vi "Pilot Analyze.vi"(5 "JoystickDevRef":T1) -> (2 "Suction":bool, 3 "x":dbl, 4 "y":dbl, 8 "Canenet L":dbl, 10 "Canenet R":dbl, 13 "Give copilot control rotation":bool, 15 "Slow Drive":bool)   [LabVIEW 2012]
uses:
  <vilib>/Rock Robotics/WPI/Joystick/WPI_JoystickDevRef.ctl
  <vilib>/Rock Robotics/WPI/Joystick/WPI_JoystickDeviceEnum.ctl
panel:
  out "Feeder":bool
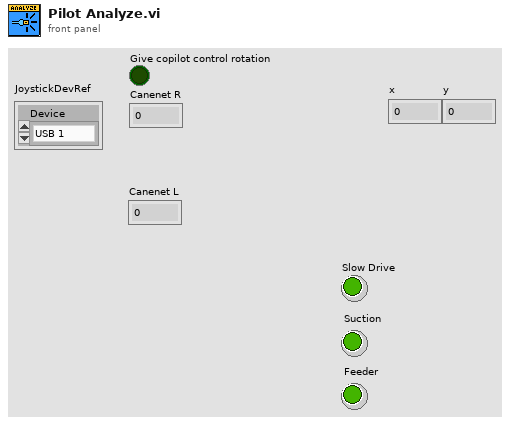
[diagram p1: front panel]
types:
  T1 = typedef "WPI_JoystickDevRef.ctl" = cluster{"Device":T2}
  T2 = typedef "WPI_JoystickDeviceEnum.ctl" = enum16{"USB 1", "USB 2", "USB 3", "USB 4", "Kinect 1", "Kinect 2"}
  T3 = typedef "WPI_JoystickButtonState.ctl" = cluster{"Button 1":bool, "Button 2":bool, "Button 3":bool, "Button 4":bool, "Button 5":bool, "Button 6":bool, "Button 7":bool, "Button 8":bool, "Button 9":bool, "Button 10":bool, "Button 11":bool, "Button 12":bool}
  T4 = cluster{"axis 1 (x)":dbl, "axis 2 (y)":dbl, "axis 3 (throttle)":dbl, "axis 4":dbl, "axis 5":dbl, "axis 6":dbl}
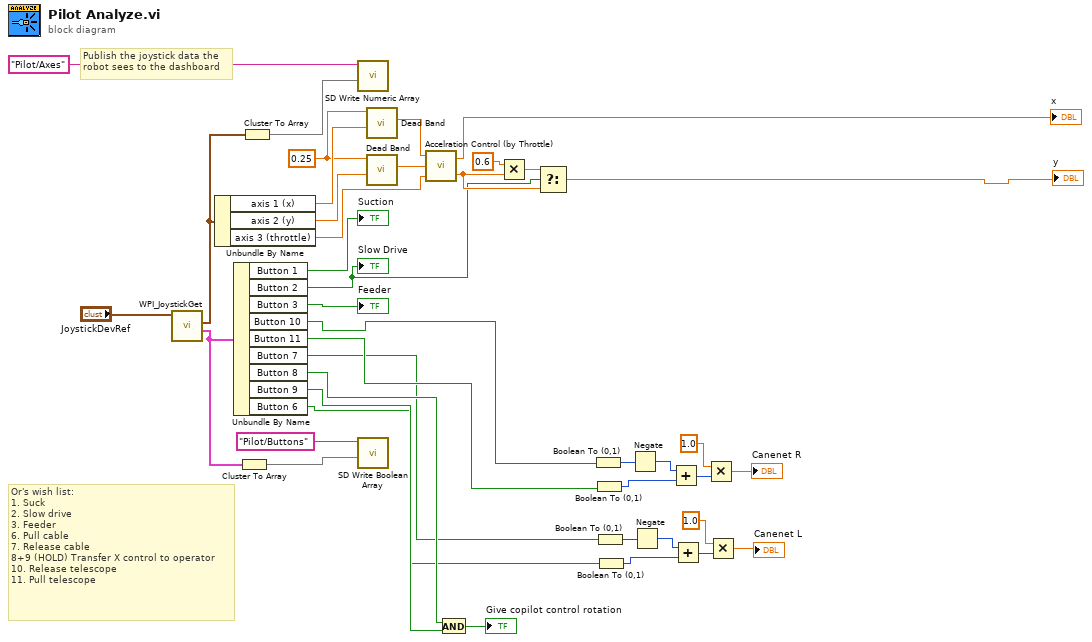
[diagram p0: block diagram]
diagram:
  w35 = 0.25 ("Dead Band")
  # "Or's wish list:\n1. Suck\n2. Slow drive\n3. Feeder\n6. Pull cable\n7. Release cable \n8+9 (HOLD) Transfer X control to operator\n10. Release telescope\n11. Pull telescope"
  # "Publish the joystick data the\nrobot sees to the dashboard"
  n1 = call <vilib>:"WPI_JoystickGet.vi"("JoystickDevRef"="JoystickDevRef") -> ("Buttons"=w29:T3, "Axes"=w30:T4)  [unwired: 4 in, 1 out]
  n2 = Unbundle By Name(w30) -> ("axis 1 (x)"=w39:dbl, "axis 2 (y)"=w37:dbl, "axis 3 (throttle)"=w28:dbl)
  n3 = Unbundle By Name(w29) -> ("Button 1"=→"Suction":bool, "Button 2"=w25:bool, "Button 3"=→"Feeder":bool, "Button 10"=w18:bool, "Button 11"=w17:bool, "Button 7"=w3:bool, "Button 8"=w21:bool, "Button 9"=w20:bool, "Button 6"=w2:bool)
  "Slow Drive" <- w25
  n4 = Cluster To Array(cluster=w29) -> (array=w22:bool[])
  n5 = Cluster To Array(cluster=w30) -> (array=w32:dbl[])
  n6 = call <vilib>:"SD Write Numeric Array.vi"("Numeric Array"=w32, "Name"="Pilot/Axes") -> ()  [unwired: 8 in, 2 out]
  n7 = call <vilib>:"SD Write Boolean Array.vi"("Boolean Array"=w22, "Name"="Pilot/Buttons") -> ()  [unwired: 8 in, 2 out]
  n8 = call "Dead Band.vi"("Axis In"=w39, "Dead Band"=w35) -> ("Axis Out"=w38:dbl)  [unwired: 9 in]
  n9 = call "Dead Band.vi"("Axis In"=w37, "Dead Band"=w35) -> ("Axis Out"=w36:dbl)  [unwired: 9 in]
  n10 = call "Accelration Control (by Throttle).vi"("acc"=w28, "Yinput"=w36, "Xinput"=w38) -> ("Youtput"=w26:dbl, "Xoutput"=→"x":dbl)
  n11 = And(x=w21, y=w20) -> (x .and. y?=→"Give copilot control rotation":bool)
  n12 = Multiply(x=0.6 ("y"), y=w26) -> (x*y=w34:dbl)
  n13 = Select(t=w34, s=w25, f=w26) -> (s? t:f=→"y":dbl)
  n14 = Boolean To (0,1)(Boolean=w18) -> (0, 1=w16:i16)
  n15 = Boolean To (0,1)(Boolean=w17) -> (0, 1=w14:i16)
  n16 = Boolean To (0,1)(Boolean=w3) -> (0, 1=w4:i16)
  n17 = Boolean To (0,1)(Boolean=w2) -> (0, 1=w6:i16)
  n18 = Negate(x=w16) -> (-x=w15:i16)
  n19 = Negate(x=w4) -> (-x=w5:i16)
  n20 = Add(x=w15, y=w14) -> (x+y=w11:i16)
  n21 = Add(x=w5, y=w6) -> (x+y=w7:i16)
  n22 = Multiply(x=1.0, y=w11) -> (x*y=→"Canenet R":dbl)
  n23 = Multiply(x=1.0, y=w7) -> (x*y=→"Canenet L":dbl)
